vi "Update Fan Status.vi"(8 "error in (no error)":errorcluster, 9 "Fan B":cluster{"State":bool, "Fault":bool}, 10 "Fan A":cluster{"State":bool, "Fault":bool}, 11 "Cooler in":refnum<class "Cooler.lvclass">) -> (0 "error out":errorcluster, 3 "Cooler out":refnum<class "Cooler.lvclass">)   [LabVIEW 2015, in "Cooler.lvlib" / "Cooler.lvclass"]
uses:
  Cooler.lvclass
  Cooler.lvclass/Cooler.ctl
  Cooler UI/Cooler UI with Events Messages/Message Update Fan/Message Update Fan.lvclass/Message Update Fan.ctl
  <vilib>/ActorFramework/Message Enqueuer/Message Enqueuer.lvclass/Message Enqueuer.ctl
  <vilib>/ActorFramework/Message Enqueuer/Enqueue.vi
  <vilib>/ActorFramework/Message Priority Queue/Priority Enqueue.vi
  Cooler UI/Cooler UI with Events Messages/Message Update Fan/Message Update Fan.lvclass
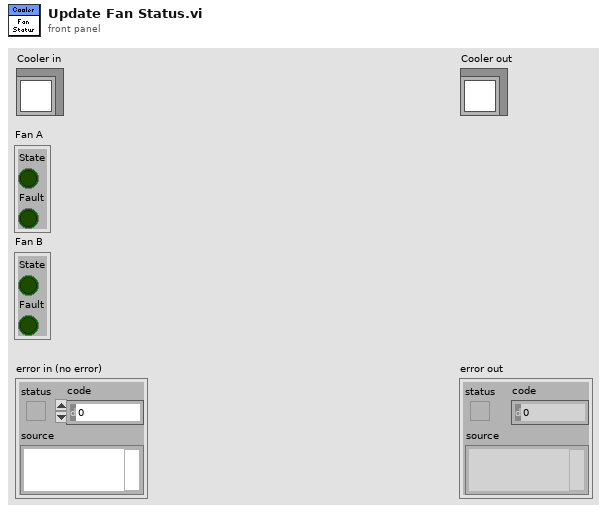
[diagram p1: front panel]
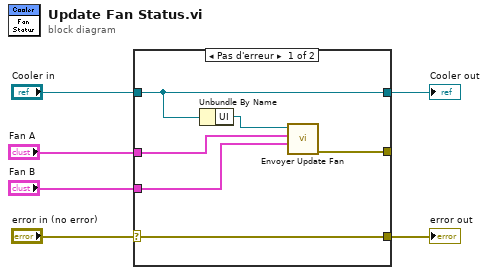
[diagram p0: block diagram]
diagram:
  n1 = case shown="Pas d'erreur" "error in (no error)" {
    selector: "error in (no error)" -> [w12 w14]
    tunnel: [w12 w14] -> w5
    tunnel: [w11 w13] -> w3
    tunnel: "Cooler in" -> [w11 w13]
    tunnel: "Fan A" -> [w9 _]
    tunnel: "Fan B" -> [w8 _]
    tunnel: [w7 _] -> _
    frame No Error {
      n2 = Unbundle By Name(w11) -> ("UI"=w10:refnum<class "Message Enqueuer.lvclass">)
      n3 = call "Envoyer Update Fan.vi"("Fan B"=w8, "Fan A"=w9, "Message Enqueuer"=w10) -> ("error out"=w7:errorcluster)  [unwired: 7 in, 1 out]
    }
    frame Error {
    }
  }
  "error out" <- w5
  "Cooler out" <- w3
